vi "List VIs without Test Coverage.vi"(8 "error in (no error)":errorcluster, 10 "Source Root":path) -> (0 "error out":errorcluster, 2 "VIs without test coverage":string[](array[string]))   [LabVIEW 2009]
uses:
  <userlib>/_OpenG.lib/array/array.llb/Conditional Auto-Indexing Tunnel (String)__ogtk.vi
  <userlib>/_OpenG.lib/file/file.llb/Compare Two Paths - Scalar__ogtk.vi
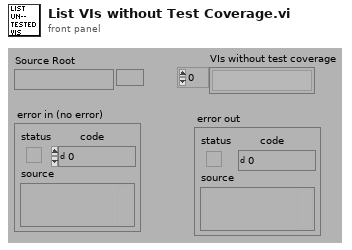
[diagram p1: front panel]
types:
  T1 = cluster{"Standard VIs":string[], "Control Type Definitions":string[], "Global VIs":string[], "Polymorphic VIs":string[]}
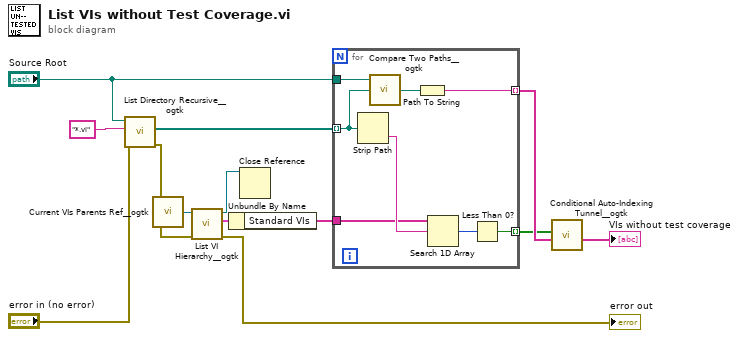
[diagram p0: block diagram]
diagram:
  n1 = call <userlib>:"List Directory Recursive__ogtk.vi"("error in (no error)"="error in (no error)", "pattern"="*.vi", "Path"="Source Root") -> ("error out"=w10:errorcluster, "file paths"=w8:path[])  [unwired: 5 in, 2 out]
  n2 = call <userlib>:"Current VIs Parents Ref__ogtk.vi"() -> ("Calling VI's reference"=w2:refnum<vi>)  [unwired: 2 in]
  n3 = call <userlib>:"List VI Hierarchy__ogtk.vi"("error in (no error)"=w10, "VI reference"=w2) -> ("error out"=→"error out":errorcluster, "Hierarchy Lists"=w3:T1, "dup VI reference"=w13:refnum<vi>)  [unwired: 7 in]
  n4 = Unbundle By Name(w3) -> ("Standard VIs"=w4:string[])
  n5 = Close Reference(reference=w13) -> ()  [unwired: 1 in, 1 out]
  n6 = for {
    tunnel: w8 -> [w16] mode=indexing
    tunnel: w4 -> [w20]
    tunnel: [w18] -> w5 mode=indexing
    tunnel: "Source Root" -> [w17]
    tunnel: [w14] -> w7 mode=indexing
    n7 = Strip Path(path=w16) -> (name=w21:string)  [unwired: 1 out]
    n8 = call-poly <userlib>:"Compare Two Paths__ogtk.vi"("path2"=w16, "path1"=w17) -> ("relative path from 1 to 2"=w15:path)  [unwired: 1 in, 2 out]
    n9 = Path To String(path=w15) -> (string=w14:string)
    n10 = Search 1D Array(1D array=w20, element=w21) -> (index of element=w19:i32)  [unwired: 1 in]
    n11 = Less Than 0?(x=w19) -> (x < 0?=w18:bool)
  }
  n12 = call-poly <userlib>:"Conditional Auto-Indexing Tunnel__ogtk.vi"("Array in"=w7, "Elements to keep"=w5) -> ("Filtered Array out"=→"VIs without test coverage":string[])  [unwired: 5 in]
